vi "VA CoAP - Message - Option Insert - Generic.vi"(8 "CoAP Message IN":string="CoAP Message IN", 9 "New Message Element":string="New Message Element", 10 "Current Delta on Evaluation":u8, 11 "Current Option Delta in":u8) -> (0 "CoAP Message OUT":string, 3 "Current Option Delta out":u8)   [LabVIEW 2020]
panel:
  out "x .or. y?":bool[](array[boolean])
  out "Message Length":bool[](array[boolean])
  out "Delta Option":bool[](array[boolean])
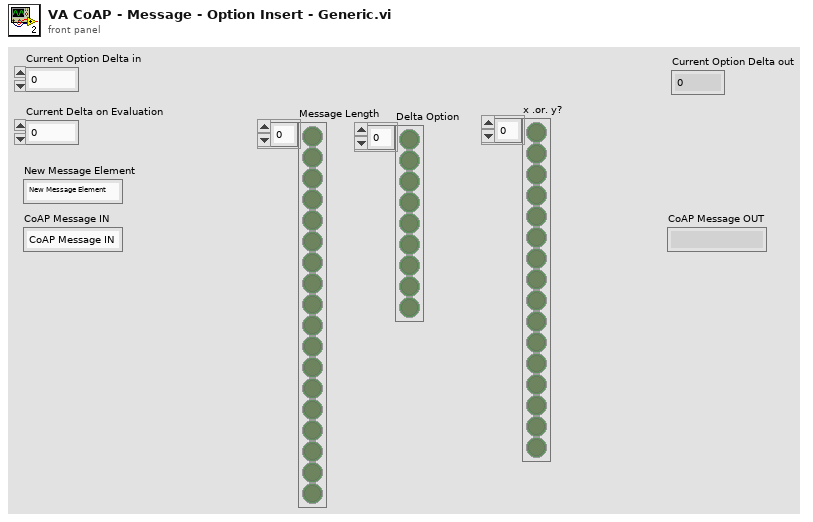
[diagram p1: front panel]
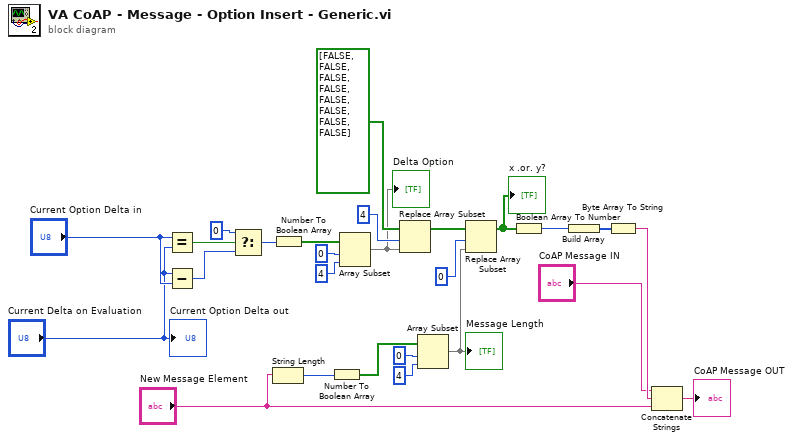
[diagram p0: block diagram]
diagram:
  n1 = Equal?(x="Current Option Delta in", y="Current Delta on Evaluation") -> (x = y?=w25:bool)
  n2 = Subtract(x="Current Delta on Evaluation", y="Current Option Delta in") -> (x-y=w26:u8)
  n3 = Select(t=u8 0, s=w25, f=w26) -> (s? t:f=w17:u8)
  n4 = String Length(string="New Message Element") -> (length=w22:i32)
  n5 = Number To Boolean Array(number=w17) -> (Boolean array=w7:bool[])
  n6 = Number To Boolean Array(number=w22) -> (Boolean array=w15:bool[])
  n7 = Array Subset(array=w7, index=0, length=4) -> (w3:bool[])
  "Delta Option" <- w3
  n8 = Replace Array Subset(array=bool[] [FALSE, FALSE, FALSE, FALSE, FALSE, FALSE, FALSE, FALSE], new element=w3, index=4) -> (w4:bool[])
  n9 = Array Subset(array=w15, index=0, length=4) -> (w11:bool[])
  "Message Length" <- w11
  n10 = Replace Array Subset(array=w4, new element=w11, index=0) -> (w12:bool[])
  "x .or. y?" <- w12
  n11 = Boolean Array To Number(Boolean array=w12) -> (number=w23:u32)
  n12 = Build Array(w23) -> (w24:u32[])
  n13 = Byte Array To String(unsigned byte array=w24) -> (string=w21:string)
  n14 = Concatenate Strings("CoAP Message IN", w21, "New Message Element") -> (→"CoAP Message OUT":string)
  "Current Option Delta out" <- "Current Delta on Evaluation"
